vi "Flush.vi"(8 "error in (no error)":errorcluster, 11 "FileStream in":refnum<class "FileStream.lvclass">) -> (0 "error out":errorcluster, 3 "FileStream out":refnum<class "FileStream.lvclass">)   [LabVIEW 2020, in "IO.lvlib" / "FileStream.lvclass"]
uses:
  FileStream.lvclass
  FileStream.lvclass/FileStream.ctl
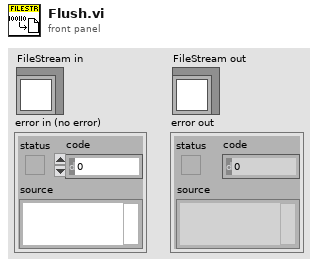
[diagram p1: front panel]
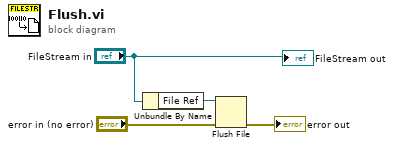
[diagram p0: block diagram]
diagram:
  n1 = Unbundle By Name("FileStream in") -> ("File Ref"=w2:refnum<file>)
  n2 = Flush File(refnum=w2, error in="error in (no error)") -> (error out=→"error out":errorcluster)  [unwired: 1 out]
  "FileStream out" <- "FileStream in"
